vi "Create File.vi"(8 "error in":errorcluster, 11 "CSV in":refnum<class "CSV.lvclass">) -> (0 "error out":errorcluster, 3 "CSV out":refnum<class "CSV.lvclass">)   [LabVIEW 2017, in "Report_lib.lvlib" / "CSV.lvclass"]
doc: "This Dynamic method uses for replace such method \nin parent class and create/replace new text file"
uses:
  CSV.lvclass
  CSV.lvclass/CSV.ctl
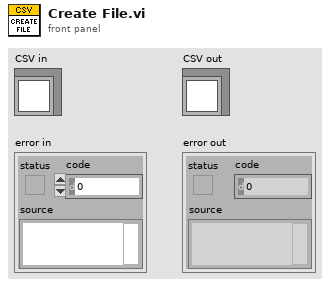
[diagram p1: front panel]
types:
  T1 = enum16{"open", "replace", "create", "open or create", "replace or create", "replace or create with confirmation"}
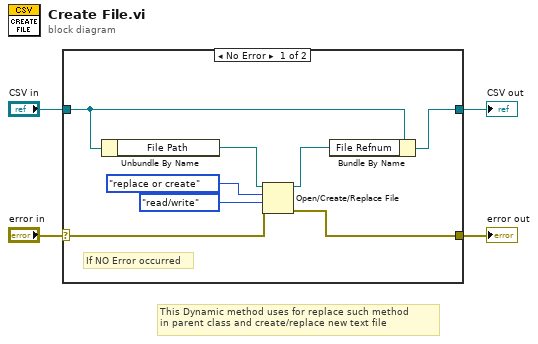
[diagram p0: block diagram]
diagram:
  # "This Dynamic method uses for replace such method \nin parent class and create/replace new text file"
  n1 = case shown="No Error" "error in" {
    selector: "error in" -> [w10 w14]
    tunnel: [w9 w14] -> w3
    tunnel: [w5 w13] -> w1
    tunnel: "CSV in" -> [w6 w13]
    frame No Error {
      # "If NO Error occurred"
      n2 = Unbundle By Name(w6) -> ("File Path"=w8:path)
      n3 = Open/Create/Replace File(file path (use dialog)=w8, error in=w10, operation (0:open)=T1."replace or create", access (0:read/write)=enum16{"read/write", "read-only", "write-only"}."read/write") -> (refnum out=w7:refnum<file>, error out=w9:errorcluster)  [unwired: 2 in, 1 out]
      n4 = Bundle By Name(cluster=w6, "File Refnum"=w7) -> (w5:refnum<class "CSV.lvclass">)
    }
    frame Error {
    }
  }
  "error out" <- w3
  "CSV out" <- w1
